vi "Create Generic 2 Queues.vi"(8 "error in (no error)":errorcluster, 11 "name":string="selectspectrum") -> (0 "error out":errorcluster, 3 "Message Queues":T1)   [LabVIEW 2022 SP3, in "Front Panel Message Queue.lvlib"]
doc: "This VI creates and initializes all the message queues for your application. If your application requires more than one message queue, right-click the \"Message Queues\" constant above and select Open Type Def. Add the new Message Queue(s) to the type definition, then initialize them in this VI."
uses:
  Front Panel Message Queue.lvlib
  Enqueue Message (Single).vi
  Message Cluster.ctl
  load 2 Messages Queues.ctl
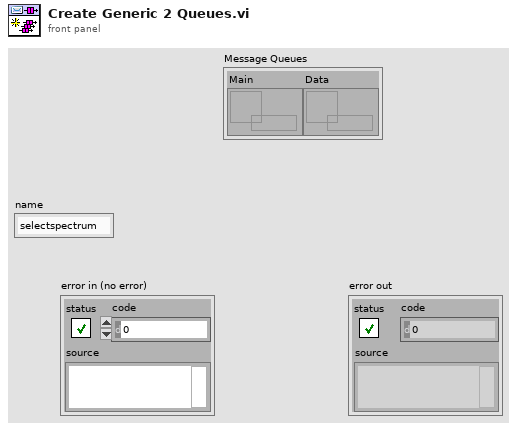
[diagram p1: front panel]
types:
  T1 = typedef "Front Panel Message Queue.lvlib/load 2 Messages Queues.ctl" = cluster{"Main":refnum<queue>, "Data":refnum<queue>}
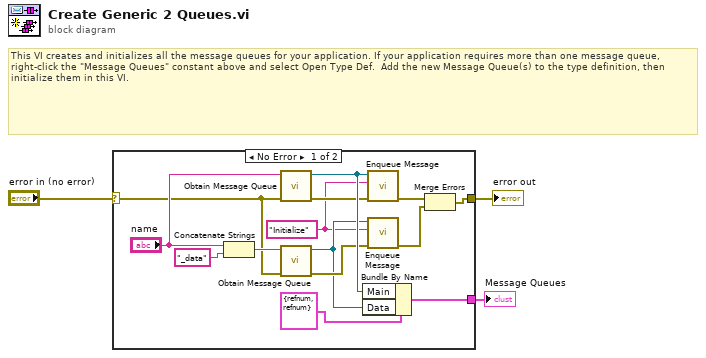
[diagram p0: block diagram]
diagram:
  # "This VI creates and initializes all the message queues for your application. If your application requires more than one message queue, right-click the \"Message Queues\" constant above and select Open Type Def.  Add the new Message Queue(s) to the type definition, then initialize them in this VI."
  n1 = case shown="No Error" "error in (no error)" {
    selector: "error in (no error)" -> [w10 w18]
    tunnel: [w7 w18] -> w3
    tunnel: [w17 _] -> w1
    frame No Error {
      w4 = "Initialize" ("Message")
      n2 = Concatenate Strings("name", "_data" ("string")) -> (w11:string)
      n3 = call "Obtain Message Queue.vi"("error in (no error)"=w10, "name"="name") -> ("error out"=w12:errorcluster, "Message Queue"=w13:refnum<queue>)  [unwired: 8 in]
      n4 = call "Obtain Message Queue.vi"("error in (no error)"=w10, "name"=w11) -> ("error out"=w9:errorcluster, "Message Queue"=w5:refnum<queue>)  [unwired: 8 in]
      n5 = Bundle By Name(cluster=T1 {"Main"=refnum, "Data"=refnum} ("Message Queues"), "Main"=w13, "Data"=w5) -> (w17:T1)
      n6 = call-poly "Enqueue Message.vi"("error in (no error)"=w12, "Message"=w4, "Message Queue"=w13) -> ("error out"=w8:errorcluster)  [unwired: 7 in, 1 out]
      n7 = call-poly "Enqueue Message.vi"("error in (no error)"=w9, "Message"=w4, "Message Queue"=w5) -> ("error out"=w6:errorcluster)  [unwired: 7 in, 1 out]
      n8 = Merge Errors(w8, w6) -> (w7:errorcluster)
    }
    frame Error {
    }
  }
  "error out" <- w3
  "Message Queues" <- w1
